vi "Find baudrate.vi"(0 "System no.":i32=1 min=1 step=1, 1 "Termination character":T1, 2 "RS-232 Portnumber":i32(ring) items=["COM1", "COM2", "COM3", "COM4", "COM5", "COM6", "COM7", "COM8", "COM9", "COM10", "COM11", "COM12", "COM13", "COM14", "COM15", "COM16", "COM17", "COM18", "COM19", "COM20", "COM21", "COM22", "COM23", "COM24", "COM25", "COM26", "COM27", "COM28", "COM29", "COM30"], 3 "Valid Baudrates":u32[](array[numeric])=[115200, 57600, 38400, 19200, 9600, 230400, 460800], 5 "error in":errorcluster, 6 "Interface clear":string="XXX\n", 7 "Bit settings and parity":T2={"data bits"=8, "stop bits"=enum."1 bit", "parity"=enum."no parity"} {"data bits" min=5 max=8 step=1}, 8 "String to Send":string="*idn?", 9 "Flow control":T3={"input XON/XOFF"=FALSE, "input HW Handshake"=FALSE, "input alt HW HShk"=FALSE, "output XON/XOFF"=FALSE, "output HW Handshake"=FALSE, "output alt HW HShk"=FALSE, "XOFF byte "=19, "XON byte"=17, "parity error byte"=0} {"parity error byte" format="%.0x"; "XON byte" format="%.0x"; "XOFF byte" format="%.0x"}, 11 "Timeout":i32=2000) -> (14 "Baudrate out":u32=115200, 15 "String read":string, 19 "error out":errorcluster)   [LabVIEW 2020]
doc: "Opens COM port of given system with valid baud rates until status of Error out is false.\n\nC-413: Input and output HW handshake must be TRUE. All other controls = default.\nC-702: Input and output HW handshake must be TRUE. All other controls = default.\nC-848: Input and output HW handshake must be TRUE. All other controls = default.\nC-867: Input and output HW handshake must be FALSE. All other controls = default. The baud rate is set via the DIP switches on the controller front panel. See the controller user manual for details.\nC-877: Input and output HW handshake must be FALSE. All other controls = default. Check controller user manual for supported baud rates.\nC-880: Input and output HW handshake must be TRUE. All other controls = default.\nC-880K005: All controls = default.\nC-884: Input and output HW handshake must be TRUE. All other controls = default. The baud rate is set via IFC/IFS.vi. See the controller user manual for details.\nC-891: Input and output HW handshake must be FALSE. All other controls = default.\nE-135: Input and output HW handshake must be TRUE. All other controls = default.\nE-516: Input and output HW handshake must be TRUE. All other controls = default.\nE-517: Input and output HW handshake must be TRUE. Not available for Interface = GPIB, TCP/IP or DLL (USB). All other controls = default.\nE-518: Input and output HW handshake must be TRUE. Not available for Interface = TCP/IP or DLL (USB). All other controls = default.\nE-709: Input and output HW handshake must be TRUE. Not available for Interface = USB. All other controls = default.\nE-712: Input and output HW handshake must be TRUE. Not available for Interface = TCP/IP or DLL. All other controls = default.\nE-725, E-727: Input and output HW handshake must be TRUE. Not available for Interface = TCP/IP or DLL (USB). All other controls = default.\nE-753: Input and output HW handshake must be TRUE. Not available for Interface = TCP/IP. All other controls = default.\nE-754: Input and output HW handshake must be TRUE. Not available for Interface = TCP/IP or DLL. All other controls = default.\nE-755: Input and output HW handshake must be TRUE. Not available for Interface = DLL and DLL Interface = RS232DC (DaisyChain). Interface clear = \\18 (Use \"\\\"Codes Display\" to enter), String to Send = err?. All other controls = default.\nE-816: Input and output HW handshake must be TRUE. All other controls = default.\nE-861: Input and output HW handshake must be FALSE. All other controls = default. The baud rate is set via the DIP switches on the controller front panel. See the E-861 user manual for details.\nE-871: Input and output HW handshake must be FALSE. All other controls = default. The baud rate is set via the DIP switches on the controller front panel. See the controller user manual for details.\nE-872: Input and output HW handshake must be FALSE. All other controls = default.\nE-873: Input and output HW handshake must be FALSE. All other controls = default.\nE-874: Input and output HW handshake must be FALSE. All other controls = default.\nC-887, F-206, M-8X0: All controls = default.\nMercury_GCS: Input and output HW handshake must be FALSE. All other controls = default. The baud rate is set via the DIP switches on the controller front panel. See the controller user manual for details."
uses:
  Termination character.ctl
  Global1.vi
panel:
  # "Opens COM Port of given system with valid baudrates until status of \"Error out\" is false."
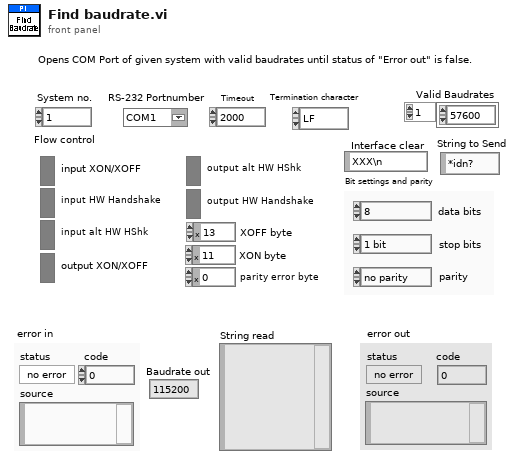
[diagram p1: front panel]
types:
  T1 = typedef "Termination character.ctl" = enum16{"LF", "CR", "LFCR", "CRLF"}
  T2 = cluster{"data bits":u16, "stop bits":enum16{"1 bit", "1.5 bits", "2 bits"}, "parity":enum16{"no parity", "odd parity", "even parity", "mark parity", "space parity"}}
  T3 = cluster{"input XON/XOFF":bool, "input HW Handshake":bool, "input alt HW HShk":bool, "output XON/XOFF":bool, "output HW Handshake":bool, "output alt HW HShk":bool, "XOFF byte ":u8, "XON byte":u8, "parity error byte":u16}
  T4 = typedef "Available interfaces.ctl" = u16
  T5 = cluster{"RS232 Portnumber":i32, "Timeout":i32, "RS232 Baud rate":u32, "Interface":T4, "GPIB Bus":i32, "GPIB Address":i32, "GPIB Mode":i32}[]
  T6 = cluster{"RS232 Portnumber":i32, "Timeout":i32, "RS232 Baud rate":u32, "Interface":T4, "GPIB Bus":i32, "GPIB Address":i32, "GPIB Mode":i32}
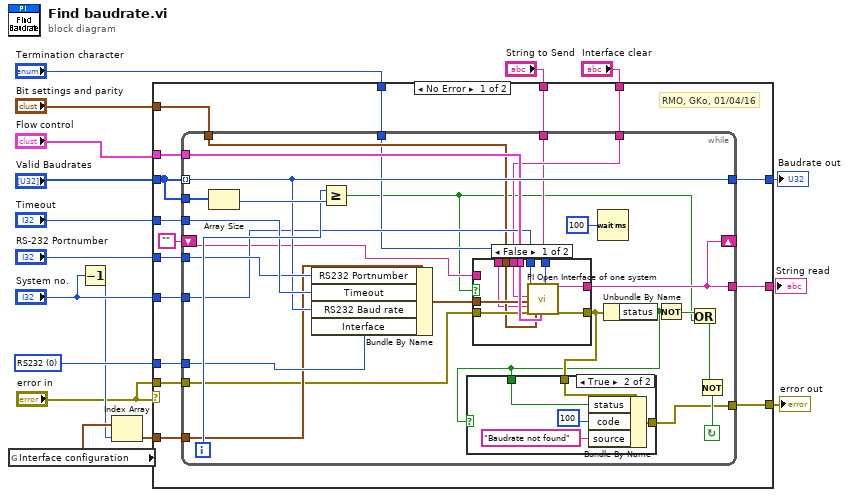
[diagram p0: block diagram]
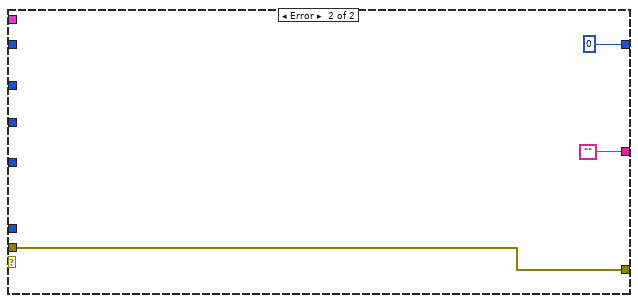
[diagram p4: hidden frame]
diagram:
  w15 = u16 0 items=["RS232", "GPIB"] ("Interface")
  n1 = global read "Global1.vi" "Interface configuration"() -> (w10:T5)
  n2 = Decrement(x="System no.") -> (x-1=w9:i32)
  n3 = Index Array(array=w10, index=w9) -> (element=w8:T6)
  n4 = case shown="No Error" "error in" {
    tunnel: "Valid Baudrates" -> [w33 _]
    tunnel: [w32 w80] -> w16
    tunnel: w15 -> [w31 _]
    tunnel: "Timeout" -> [w30 _]
    tunnel: "RS-232 Portnumber" -> [w29 _]
    tunnel: [w28 u32 0 ("Numeric")] -> w12
    tunnel: "System no." -> [w27 _]
    tunnel: "Flow control" -> [w26 _]
    tunnel: w8 -> [w25 _]
    tunnel: "error in" -> [w24 w80]
    tunnel: "Bit settings and parity" -> [w23 _]
    tunnel: "Termination character" -> [w22 _]
    tunnel: "Interface clear" -> [w21 _]
    tunnel: "String to Send" -> [w20 _]
    tunnel: [w19 ""] -> w1
    frame No Error {
      # "RMO, GKo, 01/04/16"
      n5 = while {
        tunnel: w25 -> [w43]
        tunnel: [w50] -> w28
        tunnel: w27 -> [w42]
        tunnel: [w47] -> w32
        tunnel: w31 -> [w51]
        tunnel: w29 -> [w52]
        tunnel: w30 -> [w53]
        tunnel: w33 -> [w50] mode=indexing
        tunnel: w33 -> [w59]
        tunnel: w26 -> [w45]
        tunnel: w24 -> [w41]
        tunnel: w23 -> [w40]
        tunnel: w22 -> [w39]
        tunnel: w21 -> [w38]
        tunnel: w20 -> [w37]
        tunnel: [w36] -> w19
        shift-right: [w36] -> _
        shift-left: "" ("String read") -> [w35]
        i -> [w57]
        stop <- w54 continue-if-true
        n6 = Array Size(array=w59) -> (size(s)=w58:i32)
        n7 = Bundle By Name(cluster=w43, "RS232 Portnumber"=w52, "Timeout"=w53, "RS232 Baud rate"=w50, "Interface"=w51) -> (w44:T6)
        n8 = Greater Or Equal?(x=w57, y=w58) -> (x >= y?=w34:bool)
        n9 = case shown="False" w34 {
          tunnel: [w69 w70] -> w49
          tunnel: w45 -> [w68 _]
          tunnel: w44 -> [w67 _]
          tunnel: w42 -> [w66 _]
          tunnel: w41 -> [w65 w70]
          tunnel: w40 -> [w64 _]
          tunnel: w39 -> [w63 _]
          tunnel: w38 -> [w62 _]
          tunnel: w37 -> [w61 _]
          tunnel: [w60 w71] -> w36
          tunnel: w35 -> [_ w71]
          frame False {
            n10 = call "PI Open Interface of one system.vi"("System number"=w66, "Interface clear"=w62, "Interface configuration"=w67, "String to Send"=w61, "error in"=w65, "Bit settings and parity"=w64, "Flow control"=w68, "Termination character"=w63) -> ("String read"=w60:string, "error out"=w69:errorcluster)  [unwired: 4 in, 6 out]
          }
          frame True {
          }
        }
        n11 = Wait (ms)(milliseconds to wait=u32 100) -> ()  [unwired: 1 out]
        n12 = Unbundle By Name(w49) -> ("status"=w48:bool)
        n13 = case shown="True" w48 {
          tunnel: w49 -> [w72 w77]
          tunnel: w48 -> [_ w76]
          tunnel: [w72 w73] -> w47
          frame False {
          }
          frame True {
            n14 = Bundle By Name(cluster=w77, "status"=w76, "code"=100 ("Bundle Element"), "source"="Baudrate not found" ("Bundle Element")) -> (w73:errorcluster)
          }
        }
        n15 = Not(x=w48) -> (.not. x?=w56:bool)
        n16 = Or(x=w56, y=w34) -> (x .or. y?=w55:bool)
        n17 = Not(x=w55) -> (.not. x?=w54:bool)
      }
    }
    frame Error {
    }
  }
  "error out" <- w16
  "Baudrate out" <- w12
  "String read" <- w1
